vi "Add DO Coil - Right Click.vi"() -> ()   [LabVIEW 2020, in "Modbus Master System Explorer.lvlib"]
uses:
  Modbus Master System Explorer.lvlib
  <vilib>/NI VeriStand/Custom Device API/Custom Device Item Ref.ctl
  <vilib>/NI VeriStand/Custom Device Tools/Custom Device Utility Library/Custom Device Utility Library.lvlib
  <vilib>/NI VeriStand/Custom Device API/Custom Device API.lvlib
panel:
  in  "Node Ptr":T1 format="%.0x"
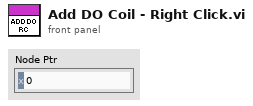
[diagram p1: front panel]
types:
  T1 = typedef "Custom Device API.lvlib/Custom Device Item Ref.ctl" = u64
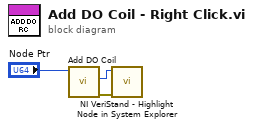
[diagram p0: block diagram]
diagram:
  n1 = call "Add DO Coil.vi"("Node Ref In"="Node Ptr") -> ("error out"=w1:errorcluster, "Channel Ref"=w2:T1)  [unwired: 8 in, 1 out]
  n2 = call <vilib>:"NI VeriStand - Highlight Node in System Explorer.vi"("error in (no error)"=w1, "Item Ref in"=w2) -> ()  [unwired: 8 in, 2 out]
